vi "2D U32 to U16.vi"(10 "Data In":u32[][](array[numeric])) -> (2 "Data Out":u16[][](array[numeric]))   [LabVIEW 2024]
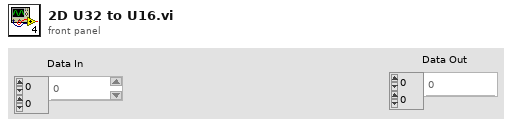
[diagram p1: front panel]
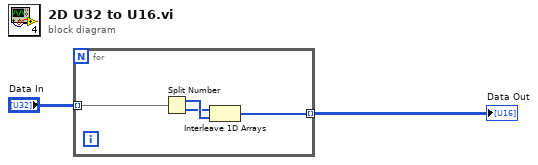
[diagram p0: block diagram]
diagram:
  n1 = for {
    tunnel: "Data In" -> [w4] mode=indexing
    tunnel: [w3] -> w1 mode=indexing
    n2 = Split Number(x=w4) -> (hi(x)=w6:u16[], lo(x)=w5:u16[])
    n3 = Interleave 1D Arrays(w5, w6) -> (w3:u16[])
  }
  "Data Out" <- w1
